vi "Read.vi"(8 "error in (no error)":errorcluster, 11 "Mettler Settings in":T1) -> (0 "error out":errorcluster, 1 "Connection Error":bool, 2 "mass (g)":dbl, 3 "Mettler Settings out":T1)   [LabVIEW 2021, in "Mettler Toledo.lvlib"]
uses:
  Mettler Toledo.lvlib
  Controls/Settings Cluster.ctl
  <vilib>/regexp/Match Regular Expression.xnode
  <vilib>/ptbypt/NI_PtbyPt.lvlib
  support/Support Library.lvlib
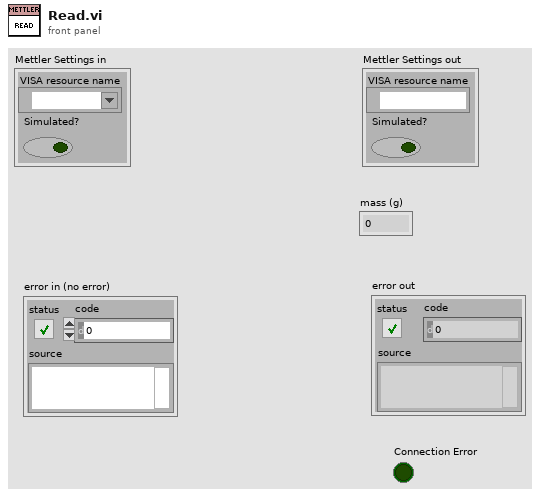
[diagram p1: front panel]
types:
  T1 = typedef "Mettler Toledo.lvlib/Settings Cluster.ctl" = cluster{"VISA resource name":refnum<visa-resource-name>, "Simulated?":bool}
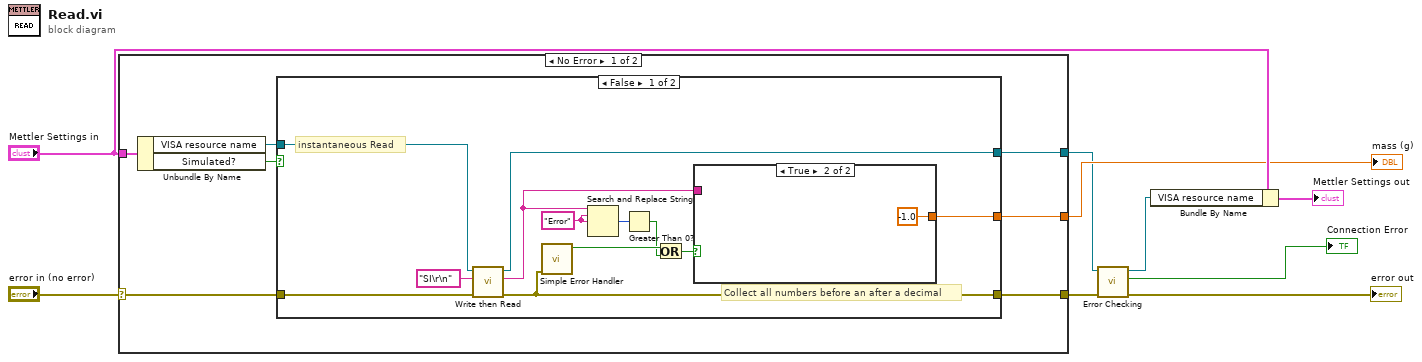
[diagram p0: block diagram]
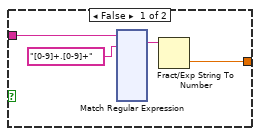
[diagram p2: hidden frame]
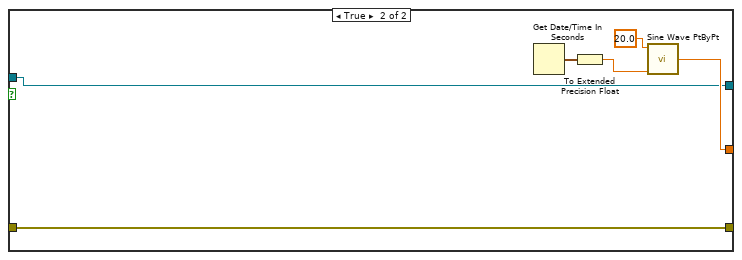
[diagram p3: hidden frame]
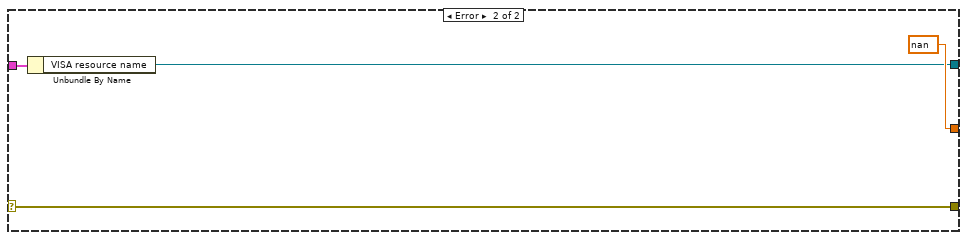
[diagram p4: hidden frame]
diagram:
  n1 = case shown="No Error" "error in (no error)" {
    selector: "error in (no error)" -> [w15 w165]
    tunnel: [w14 w165] -> w4
    tunnel: "Mettler Settings in" -> [w12 w163]
    tunnel: [w13 nan ("sine wave")] -> w7
    tunnel: [w10 w162] -> w5
    frame No Error {
      n2 = Unbundle By Name(w12) -> ("VISA resource name"=w11:refnum<visa-resource-name>, "Simulated?"=w16:bool)
      n3 = case shown="False" w16 {
        tunnel: [w23 w161] -> w14
        tunnel: w15 -> [w25 w161]
        tunnel: [w28 w157] -> w13
        tunnel: [w24 w156] -> w10
        tunnel: w11 -> [w27 w156]
        frame False {
          w19 = "Error" ("search string")
          # "Collect all numbers before an after a decimal"
          # "instantaneous Read"
          n4 = call "Write then Read.vi"("error in"=w25, "write buffer"="SI\r\n" ("Command"), "VISA resource name in"=w27) -> ("error out"=w23:errorcluster, "read buffer"=w20:string, "VISA resource name out"=w24:refnum<visa-resource-name>)  [unwired: 5 in, 1 out]
          n5 = call <vilib>:"Simple Error Handler.vi"("error in (no error)"=w23) -> ("error?"=w22:bool)  [unwired: 4 in, 4 out]
          n6 = Search and Replace String(input string=w20, search string=w19, replace string=w19) -> (number of replacements=w18:i32)  [unwired: 5 in, 3 out]
          n7 = Greater Than 0?(x=w18) -> (x > 0?=w17:bool)
          n8 = Or(x=w22, y=w17) -> (x .or. y?=w21:bool)
          n9 = case shown="True" w21 {
            tunnel: w20 -> [w31 _]
            tunnel: [w29 -1.0] -> w28
            frame False {
              n10 = xnode "Match Regular Expression"("input string"=w31, "regular expression"="[0-9]+.[0-9]+" ("Regular Expression for Extracting Weight")) -> ("whole match"=w30:string)  [unwired: 4 in, 8 out]
              n11 = Fract/Exp String To Number(string=w30) -> (number=w29:dbl)  [unwired: 3 in, 1 out]
            }
            frame True {
            }
          }
        }
        frame True {
          n12 = Get Date/Time In Seconds() -> (seconds since 1Jan1904=w160:timestamp)
          n13 = To Extended Precision Float(1:w160) -> (0:w159:ext)
          n14 = call <vilib>:"Sine Wave PtByPt.vi"("time"=w159, "amplitude"=20.0) -> ("sine wave"=w157:dbl)  [unwired: 2 in]
        }
      }
    }
    frame Error {
      n15 = Unbundle By Name(w163) -> ("VISA resource name"=w162:refnum<visa-resource-name>)
    }
  }
  "mass (g)" <- w7
  n16 = call "Error Checking.vi"("error in (no error)"=w4, "VISA resource name"=w5) -> ("error out"=→"error out":errorcluster, "Connection Error"=→"Connection Error":bool, "VISA resource name"=w2:refnum<visa-resource-name>)  [unwired: 7 in]
  n17 = Bundle By Name(cluster="Mettler Settings in", "VISA resource name"=w2) -> (→"Mettler Settings out":T1)
